vi "Main.vi"() -> ()   [LabVIEW 2025, in "Application.lvlib"]
uses:
  Application.lvlib
  Application Data--cluster.ctl
  State--enum.ctl
  <vilib>/Utility/error.llb/DialogType.ctl
  Logging - Text/Logging - Text.lvlib
  AI DAQ/AI DAQ.lvlib
panel:
  out "Waveform Graph":waveform(dbl)[](graph)
  in  "Start Acq and Log":bool
  in  "Logging File Path":path=path "C:/Users/David Corney/Documents/default log.txt"
  in  "AI DAQ Task Name":refnum<k21>="MyAnalogInTask_DiesEl"
  in  "About DQMH":bool
  out "Status":string
  out "version":string
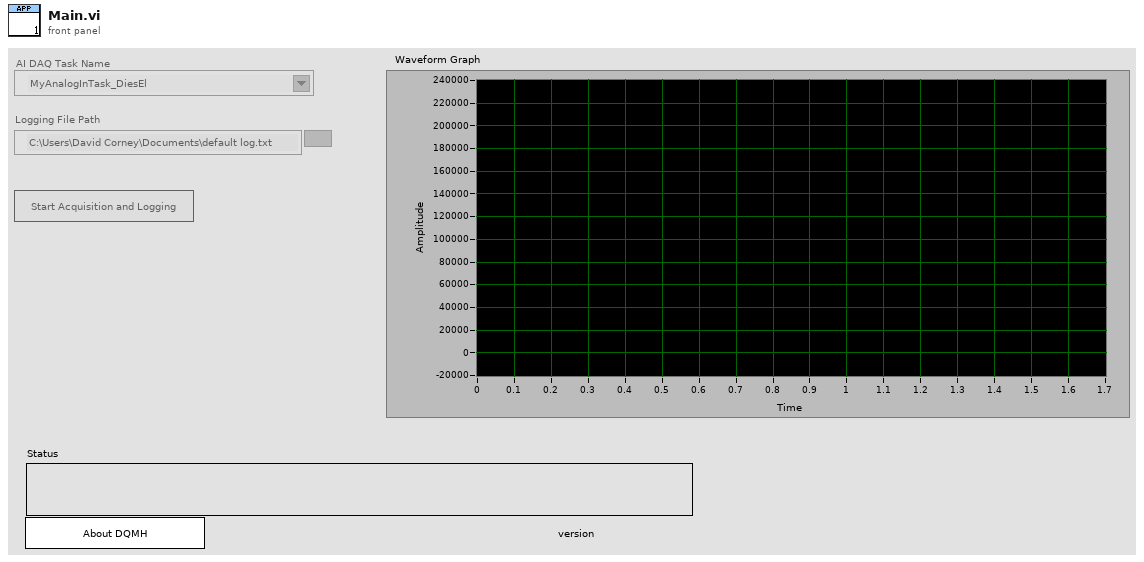
[diagram p1: front panel]
types:
  T1 = typedef "Application.lvlib/State--enum.ctl" = enum16{"Initialize", "Initialize Panel", "UI Interlocks", "Start Modules", "Update Status", "Wait for Event", "Exit"}
  T2 = typedef "Application.lvlib/Application Data--cluster.ctl" = cluster{"Status":string, "Singleton Controls":refnum<vi>[], "Cloneable Controls":refnum<vi>[], "App Controls":refnum<vi>[]}
  T3 = typedef "Logging - Text.lvlib/Broadcast Events--cluster.ctl" = cluster{"Module Did Init":refnum<user-event>, "Status Updated":refnum<user-event>, "Error Reported":refnum<user-event>, "Module Did Stop":refnum<user-event>, "Update Module Execution Status":refnum<user-event>}
  T4 = typedef "AI DAQ.lvlib/Broadcast Events--cluster.ctl" = cluster{"Module Did Init":refnum<user-event>, "Status Updated":refnum<user-event>, "Error Reported":refnum<user-event>, "Module Did Stop":refnum<user-event>, "Update Module Execution Status":refnum<user-event>, "AI DAQ WF Data":refnum<user-event>}
  T5 = enum8{"Enabled", "Disabled", "Disabled and Grayed Out"}
  T6 = typedef "DialogType.ctl" = u16
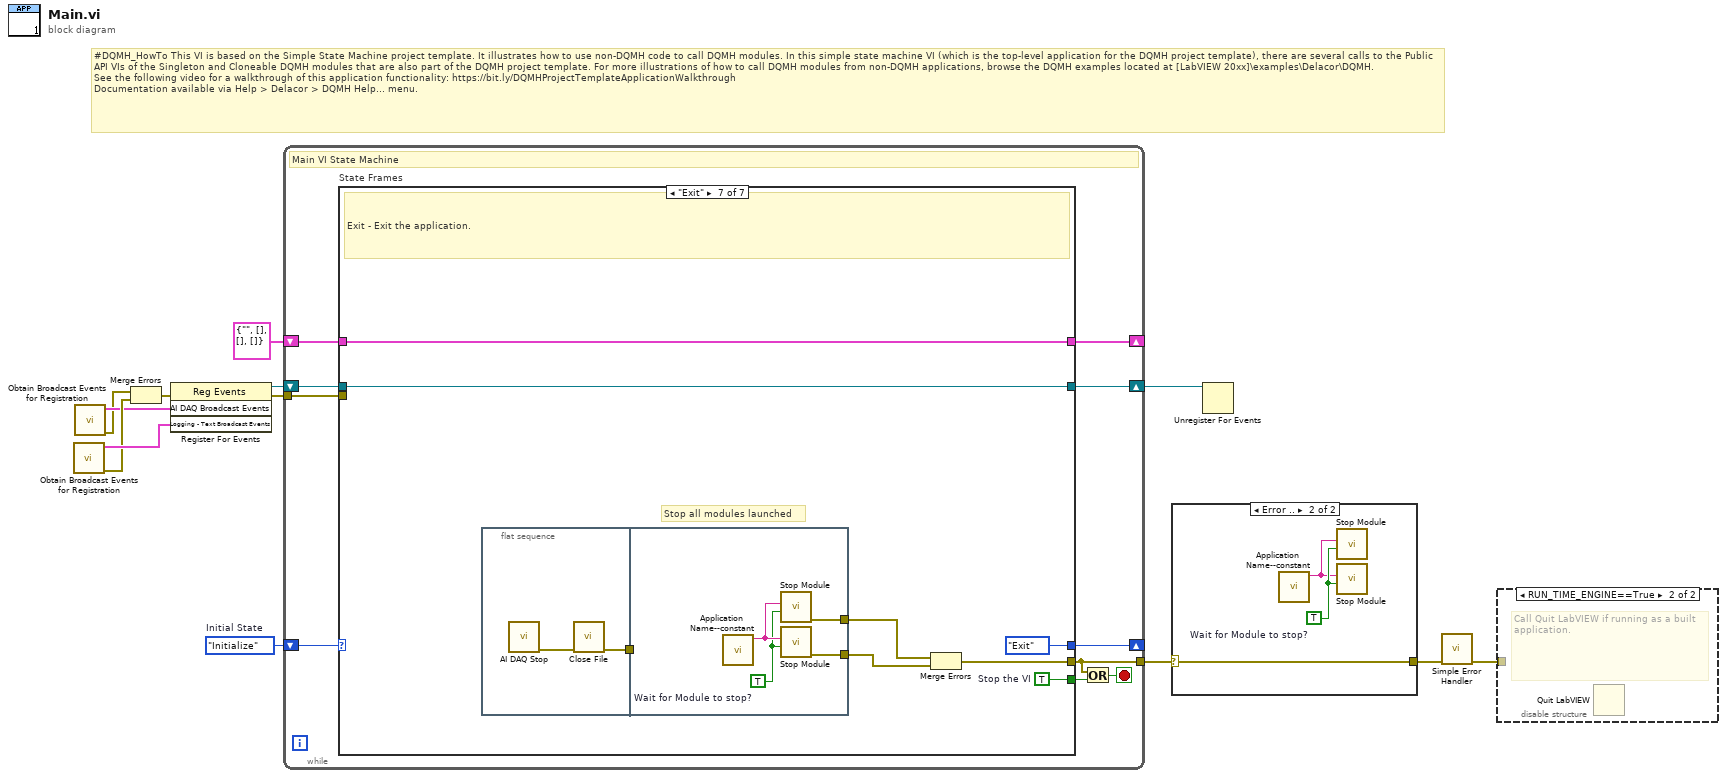
[diagram p0: block diagram]
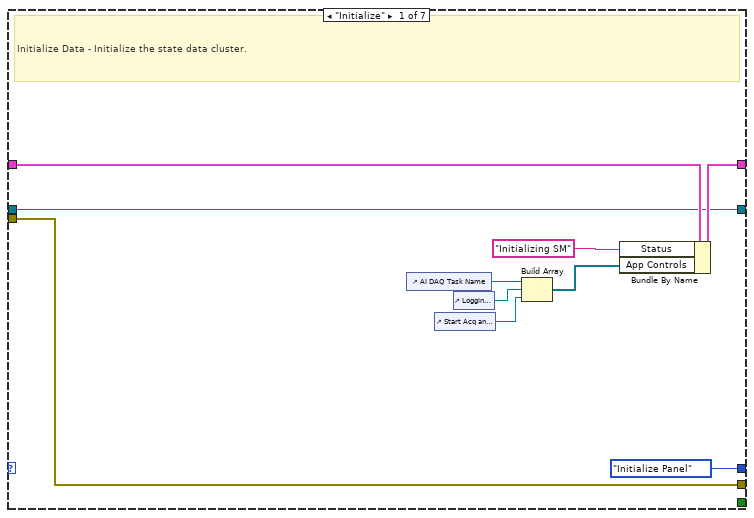
[diagram p3: hidden frame]
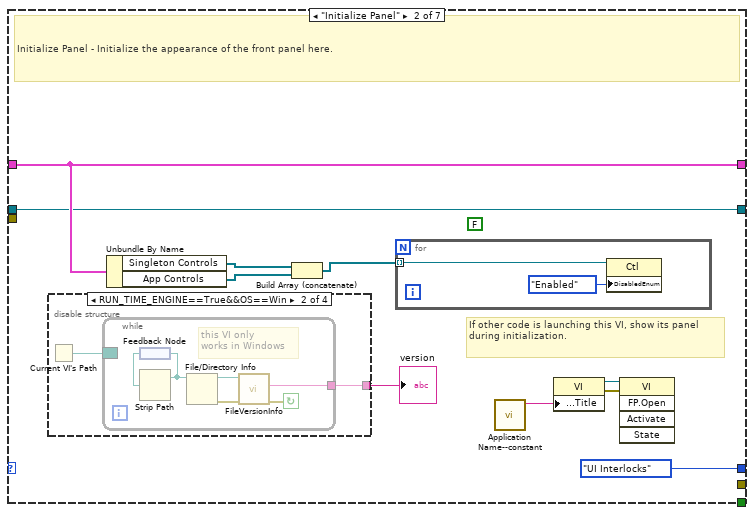
[diagram p4: hidden frame]
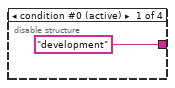
[diagram p5: hidden frame]
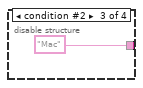
[diagram p6: hidden frame]
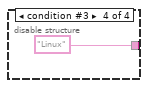
[diagram p7: hidden frame]
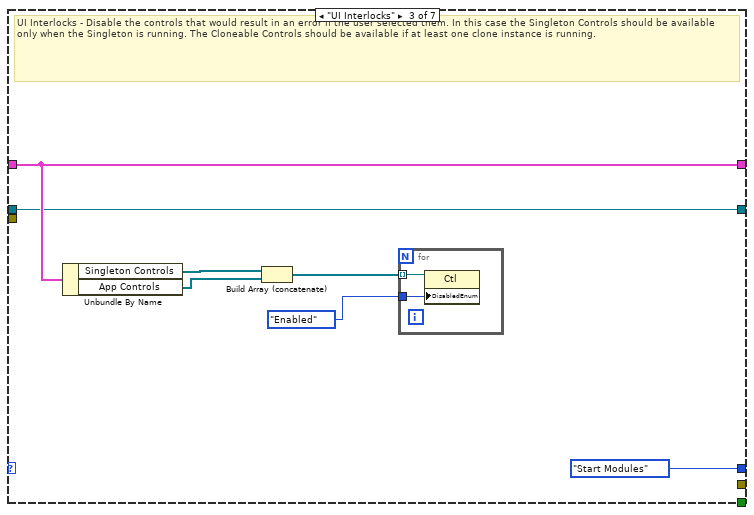
[diagram p8: hidden frame]
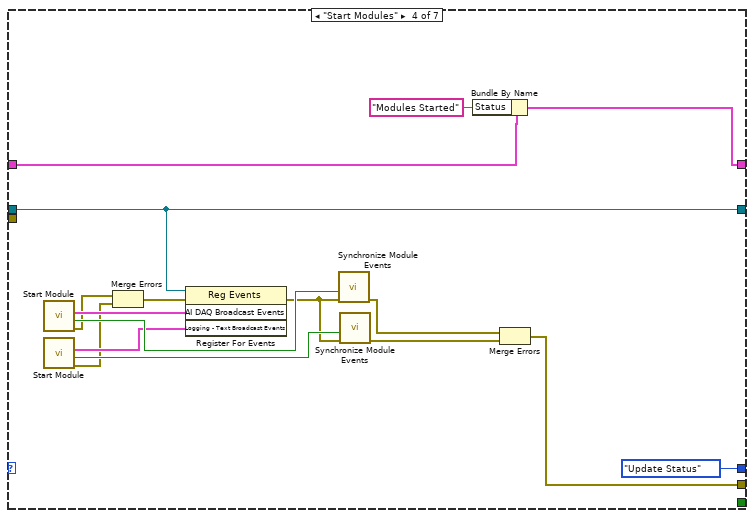
[diagram p9: hidden frame]
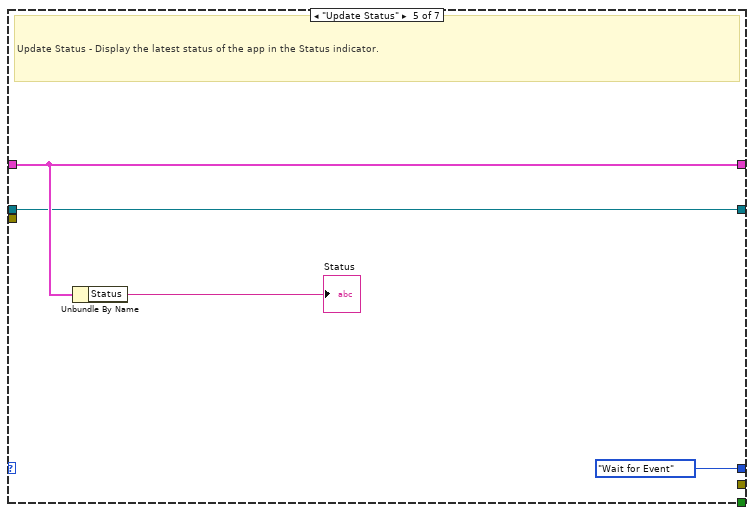
[diagram p10: hidden frame]
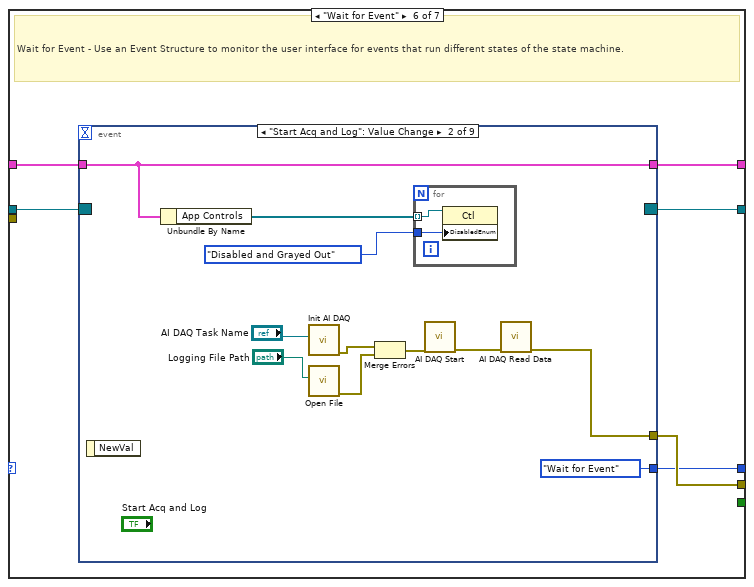
[diagram p11: hidden frame]
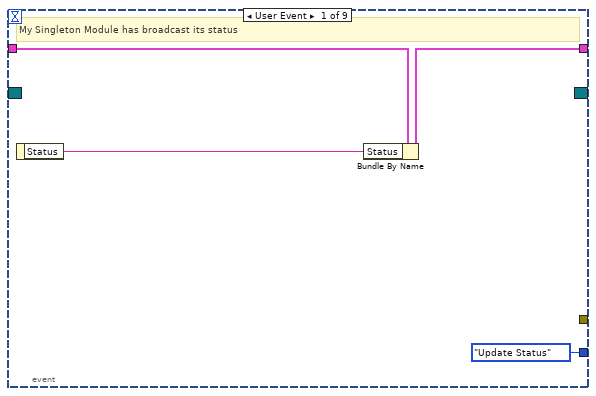
[diagram p12: hidden frame]
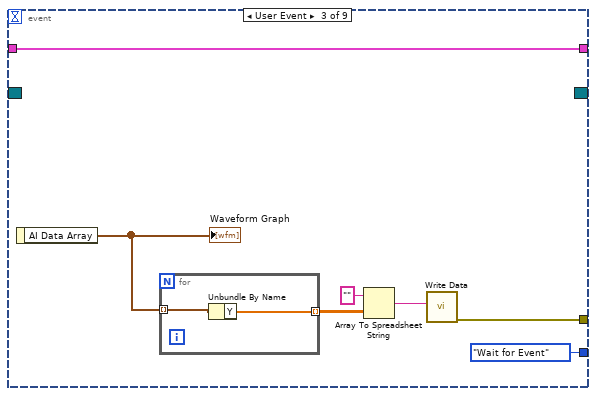
[diagram p13: hidden frame]
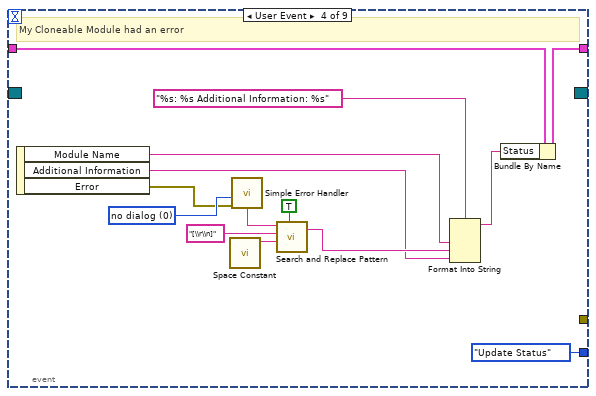
[diagram p14: hidden frame]
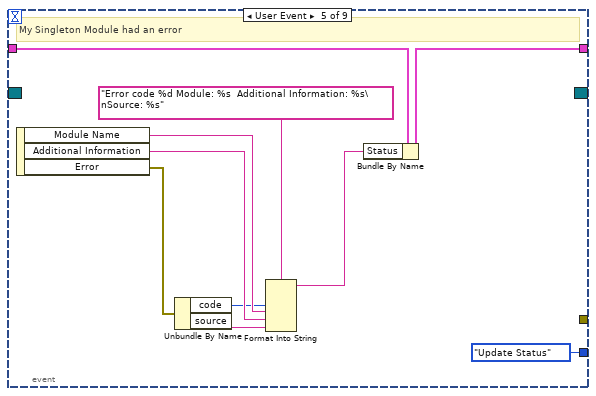
[diagram p15: hidden frame]
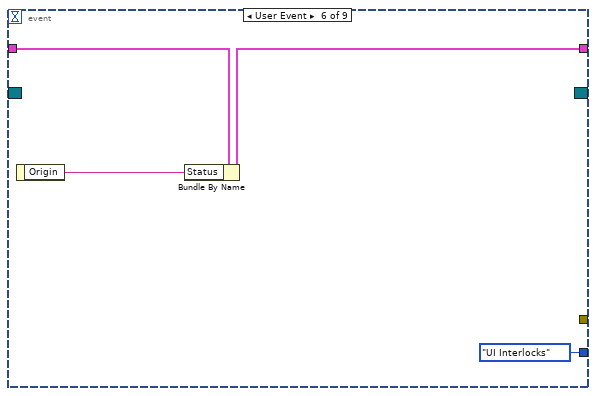
[diagram p16: hidden frame]
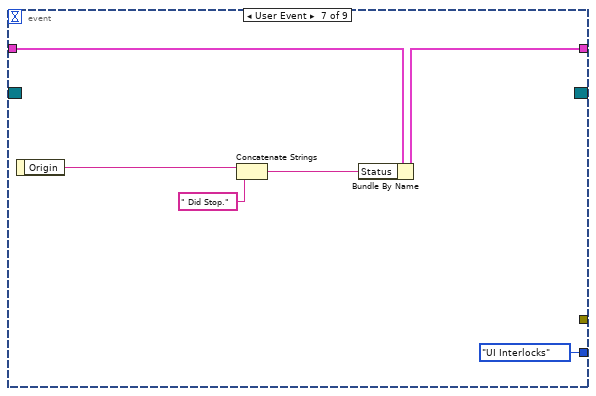
[diagram p17: hidden frame]
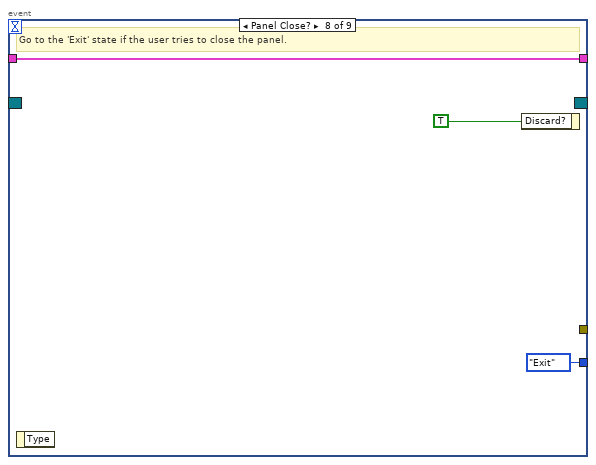
[diagram p18: hidden frame]
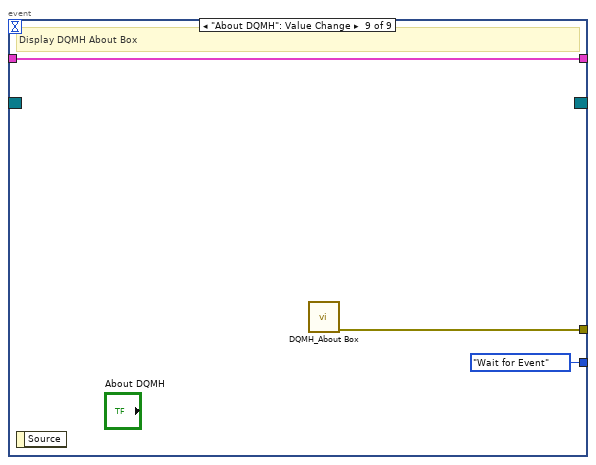
[diagram p19: hidden frame]
diagram:
  w9 = State--enum."Initialize"  # Initial State
  # "#DQMH_HowTo This VI is based on the Simple State Machine project template. It illustrates how to use non-DQMH code to call DQMH modules. In this simple state machine VI (which is the top-level application for the DQMH project template), there are several calls to the Public API VIs of the Singleton and Cloneable DQMH modules that are also part of the DQMH project template. For more illustrations of how to call DQMH modules from non-DQMH applications, browse the DQMH examples located at [LabVIEW 20xx]\\examples\\Delacor\\DQMH.\nSee the following video for a walkthrough of this application functionality: https://bit.ly/DQMHProjectTemplateApplicationWalkthrough\nDocumentation available via Help > Delacor > DQMH Help... menu."
  n1 = call "Obtain Broadcast Events for Registration.vi"() -> ("error out"=w5:errorcluster, "Logging - Text Broadcast Events"=w6:T3)  [unwired: 9 in, 1 out]
  n2 = call "Obtain Broadcast Events for Registration.vi"() -> ("error out"=w3:errorcluster, "AI DAQ Broadcast Events"=w4:T4)  [unwired: 9 in, 1 out]
  n3 = Merge Errors(w3, w5) -> (w11:errorcluster)
  n4 = register-events(error in=w11, w4, w6) -> (reference out=w8:refnum<event-registration>, error out=w12:errorcluster)  [unwired: 1 in]
  n5 = while {
    shift-right: [w20] -> _
    shift-left: T2 {"Status"="", "Singleton Controls"=[], "Cloneable Controls"=[], "App Controls"=[]} ("Data Cluster") -> [w21]
    tunnel: [w23] -> w2
    shift-right: [w16] -> _
    shift-left: w9 -> [w18]
    shift-right: [w14] -> w7
    shift-left: w8 -> [w15]
    tunnel: w12 -> [w22]
    stop <- w17 stop-if-true
    # "Main VI State Machine"
    n6 = case "State Frames" shown="\"Exit\"" w18 {
      tunnel: [w33 _ _ w71 _ w91 w165] -> w23
      tunnel: w21 -> [w32 w42 w63 w68 w85 w88 w164]
      tunnel: [w31 w42 w63 w66 w85 w87 w164] -> w20
      tunnel: [_ _ _ _ _ _ w163] -> w19
      tunnel: [State--enum."Initialize Panel" ("State") State--enum."UI Interlocks" ("State") State--enum."Start Modules" ("State") State--enum."Update Status" ("State") State--enum."Wait for Event" ("State") w86 State--enum."Exit" ("State")] -> w16
      tunnel: w15 -> [w28 w40 w61 w80 w82 w90 w161]
      tunnel: [w28 w40 w61 w80 w82 w89 w161] -> w14
      tunnel: w22 -> [w33 _ _ _ _ _ _]
      frame "Initialize" {
        # "Initialize Data - Initialize the state data cluster."
        n7 = control-ref of="AI DAQ Task Name"() -> (w26:refnum<vi>)
        n8 = control-ref of="Start Acq and Log"() -> (w24:refnum<vi>)
        n9 = control-ref of="Logging File Path"() -> (w25:refnum<vi>)
        n10 = Build Array(w26, w25, w24) -> (w27:refnum<vi>[])
        n11 = Bundle By Name(cluster=w32, "Status"="Initializing SM" ("Initial Message"), "App Controls"=w27) -> (w31:T2)
      }
      frame "Initialize Panel" {
        (unwired) FALSE ("My Singleton Module Init?")
        # "If other code is launching this VI, show its panel during initialization."
        # "Initialize Panel - Initialize the appearance of the front panel here."
        n12 = disable-structure "Conditional Disable Structure" shown="RUN_TIME_ENGINE==True&&OS==Win" {
          disable-tunnel: ["development" w45 "Mac" "Linux"] -> w39
          frame condition #0 (active) {
          }
          frame condition #1 {
            n13 = Current VI's Path() -> (path=w46:path)
            n14 = while {
              border: w46 -> [_]
              tunnel: [w47] -> w45
              stop <- w51 continue-if-true
              # "this VI only \nworks in Windows"
              n15 = feedback #1() -> (w50:path)
              n16 = Strip Path(path=w50) -> (stripped path=w49:path)  [unwired: 1 out]
              n17 = feedback-in #1(w49) -> ()
              n18 = File/Directory Info(path=w49) -> (path out=w48:path, error out=w52:errorcluster)  [unwired: 1 in, 5 out]
              n19 = call <vilib>:"FileVersionInfo.vi"("error in (no error)"=w52, "Application Path in"=w48) -> ("error out"=w51:errorcluster, "File Version Info"=w47:string)  [unwired: 6 in, 2 out]
            }
          }
          frame condition #2 {
          }
          frame condition #3 {
          }
        }
        "version" <- w39
        n20 = Unbundle By Name(w42) -> ("Singleton Controls"=w36:refnum<vi>[], "App Controls"=w35:refnum<vi>[])
        n21 = Build Array (concatenate)(w36, w35) -> (w34:refnum<vi>[])
        n22 = for {
          tunnel: w34 -> [w56] mode=indexing
          n23 = property on="Property Node" class="Ctl"(reference=w56, "DisabledEnum"=T5."Enabled" ("Disabled")) -> ()  [unwired: 1 in, 2 out]
        }
        n24 = call "Application Name--constant.vi"() -> ("Application Name"=w38:string)  [unwired: 11 in]
        n25 = property on="Property Node" class="VI"("Front Panel.Title"=w38) -> (reference out=w37:refnum<vi>, error out=w43:errorcluster)  [unwired: 2 in]
        n26 = invoke class="VI" method="FP.Open"(reference=w37, error in=w43) -> ()  [unwired: 3 in, 5 out]
      }
      frame "UI Interlocks" {
        # "UI Interlocks - Disable the controls that would result in an error if the user selected them. In this case the Singleton Controls should be available only when the Singleton is running. The Cloneable Controls should be available if at least one clone instance is running."
        n27 = Unbundle By Name(w63) -> ("Singleton Controls"=w60:refnum<vi>[], "App Controls"=w57:refnum<vi>[])
        n28 = Build Array (concatenate)(w60, w57) -> (w59:refnum<vi>[])
        n29 = for {
          tunnel: w59 -> [w65] mode=indexing
          tunnel: T5."Enabled" ("Disabled") -> [w64]
          n30 = property on="Property Node" class="Ctl"(reference=w65, "DisabledEnum"=w64) -> ()  [unwired: 1 in, 2 out]
        }
      }
      frame "Start Modules" {
        n31 = call "Start Module.vi"() -> ("error out"=w75:errorcluster, "Wait for Event Sync?"=w78:bool, "AI DAQ Broadcast Events"=w79:T4)  [unwired: 8 in, 1 out]
        n32 = call "Start Module.vi"() -> ("error out"=w74:errorcluster, "Wait for Event Sync?"=w76:bool, "Logging - Text Broadcast Events"=w77:T3)  [unwired: 8 in, 1 out]
        n33 = Merge Errors(w75, w74) -> (w73:errorcluster)
        n34 = register-events(reference=w80, error in=w73, w79, w77) -> (error out=w72:errorcluster)  [unwired: 1 out]
        n35 = call "Synchronize Module Events.vi"("error in"=w72, "Wait for Event Sync?"=w78) -> ("error out"=w70:errorcluster)  [unwired: 9 in]
        n36 = call "Synchronize Module Events.vi"("error in"=w72, "Wait for Event Sync?"=w76) -> ("error out"=w69:errorcluster)  [unwired: 9 in]
        n37 = Bundle By Name(cluster=w68, "Status"="Modules Started") -> (w66:T2)
        n38 = Merge Errors(w70, w69) -> (w71:errorcluster)
      }
      frame "Update Status" {
        # "Update Status - Display the latest status of the app in the Status indicator."
        n39 = Unbundle By Name(w85) -> ("Status"=→"Status":string)
      }
      frame "Wait for Event" {
        # "Wait for Event - Use an Event Structure to monitor the user interface for events that run different states of the state machine."
        n40 = event shown="[1] \"Start Acq and Log\": Value Change" {
          selector: w90 -> [_ _ _ _ _ _ _ _ _]
          dyn-events: [_ _ _ _ _ _ _ _ _] -> w89
          timeout: _ -> [_ _ _ _ _ _ _ _ _]
          tunnel: [_ w104 w110 _ _ _ _ _ w155] -> w91
          tunnel: [w93 w103 w115 w130 w139 w142 w149 w153 w157] -> w87
          tunnel: w88 -> [w94 w103 w115 w131 w140 w144 w150 w153 w157]
          tunnel: [State--enum."Update Status" ("State") State--enum."Wait for Event" ("State") State--enum."Wait for Event" ("State") State--enum."Update Status" ("State") State--enum."Update Status" ("State") State--enum."UI Interlocks" ("State") State--enum."UI Interlocks" ("State") State--enum."Exit" ("State") State--enum."Wait for Event" ("State")] -> w86
          event User Event {
            # "My Singleton Module has broadcast its status"
            n41 = event-data() -> ("Status"=w95:string)  [unwired: 1 in]
            n42 = Bundle By Name(cluster=w94, "Status"=w95) -> (w93:T2)
          }
          event "Start Acq and Log": Value Change {
            n43 = event-data() -> ()  [unwired: 1 in, 1 out]
            n44 = Unbundle By Name(w103) -> ("App Controls"=w96:refnum<vi>[])
            n45 = call "Init AI DAQ.vi"("AI DAQ Task Name"="AI DAQ Task Name") -> ("error out"=w98:errorcluster)  [unwired: 10 in]
            n46 = call "Open File.vi"("Path"="Logging File Path") -> ("error out"=w97:errorcluster)  [unwired: 10 in]
            n47 = Merge Errors(w98, w97) -> (w99:errorcluster)
            n48 = for {
              tunnel: T5."Disabled and Grayed Out" ("Disabled") -> [w108]
              tunnel: w96 -> [w107] mode=indexing
              n49 = property class="Ctl"(reference=w107, "DisabledEnum"=w108) -> ()  [unwired: 1 in, 2 out]
            }
            n50 = call "AI DAQ Start.vi"("error in"=w99) -> ("error out"=w105:errorcluster)  [unwired: 10 in]
            n51 = call "AI DAQ Read Data.vi"("error in"=w105) -> ("error out"=w104:errorcluster)  [unwired: 9 in, 1 out]
          }
          event User Event {
            n52 = event-data() -> ("AI Data Array"=w113:waveform(dbl)[])  [unwired: 1 in]
            "Waveform Graph" <- w113
            n53 = for {
              tunnel: w113 -> [w117] mode=indexing
              tunnel: [w116] -> w112 mode=indexing
              n54 = Unbundle By Name(w117) -> ("Y"=w116:dbl[])
            }
            n55 = Array To Spreadsheet String(array=w112, 3:"" ("format string")) -> (spreadsheet string=w111:string)  [unwired: 1 in]
            n56 = call "Write Data.vi"("Text Data"=w111) -> ("error out"=w110:errorcluster)  [unwired: 10 in]
          }
          event User Event {
            w122 = T6 0 items=["no dialog", "OK message", "continue or stop message", "OK message + warnings", "continue/stop + warnings"] ("type of dialog (OK msg:1)")
            # "My Cloneable Module had an error"
            n57 = event-data() -> ("Module Name"=w119:string, "Additional Information"=w120:string, "Error"=w121:errorcluster)  [unwired: 1 in]
            n58 = call <vilib>:"Space Constant.vi"() -> ("String"=w126:string)
            n59 = call <vilib>:"Simple Error Handler.vi"("type of dialog (OK msg:1)"=w122, "error in (no error)"=w121) -> ("message"=w123:string)  [unwired: 3 in, 4 out]
            n60 = call <vilib>:"Search and Replace Pattern.vi"("string"=w123, "regular expression (\"\")"="[\\r\\n]" ("regular expression (\"\")"), "replace string (\"\")"=w126, "replace all? (F)"=TRUE ("replace all CR/LF with spaces")) -> ("result string"=w124:string)  [unwired: 1 in, 1 out]
            n61 = Format Into String(format string="%s: %s Additional Information: %s", w119, w124, w120) -> (resulting string=w118:string)  [unwired: 2 in, 1 out]
            n62 = Bundle By Name(cluster=w131, "Status"=w118) -> (w130:T2)
          }
          event User Event {
            # "My Singleton Module had an error"
            n63 = event-data() -> ("Module Name"=w133:string, "Additional Information"=w137:string, "Error"=w141:errorcluster)  [unwired: 1 in]
            n64 = Unbundle By Name(w141) -> ("code"=w132:i32, "source"=w136:string)
            n65 = Format Into String(format string="Error code %d Module: %s  Additional Information: %s\nSource: %s", w132, w133, w137, w136) -> (resulting string=w134:string)  [unwired: 2 in, 1 out]
            n66 = Bundle By Name(cluster=w140, "Status"=w134) -> (w139:T2)
          }
          event User Event {
            n67 = event-data() -> ("Origin"=w143:string)  [unwired: 1 in]
            n68 = Bundle By Name(cluster=w144, "Status"=w143) -> (w142:T2)
          }
          event User Event {
            n69 = event-data() -> ("Origin"=w147:string)  [unwired: 1 in]
            n70 = Concatenate Strings(w147, " Did Stop.") -> (w146:string)
            n71 = Bundle By Name(cluster=w150, "Status"=w146) -> (w149:T2)
          }
          event Panel Close? {
            # "Go to the 'Exit' state if the user tries to close the panel."
            n72 = event-data() -> ()  [unwired: 1 in, 1 out]
            n73 = event-data ("Event Filter Node")("Discard?"=TRUE) -> ()  [unwired: 1 in, 1 out]
          }
          event "About DQMH": Value Change {
            # "Display DQMH About Box"
            n74 = event-data() -> ()  [unwired: 1 in, 1 out]
            n75 = call <vilib>:"DQMH_About Box.vi"() -> ("error out"=w155:errorcluster)  [unwired: 11 in]
          }
        }
      }
      frame "Exit" {
        w163 = TRUE  # Stop the VI
        # "Stop all modules launched"
        # "Exit - Exit the application."
        n76 = flat-sequence {
          tunnel: [w166] -> w158
          tunnel: [w169] -> w159
          tunnel: [w168] -> w160
          tunnel: w158 -> [_]
          frame #0 {
            n77 = call "AI DAQ Stop.vi"() -> ("error out"=w167:errorcluster)  [unwired: 11 in]
            n78 = call "Close File.vi"("error in"=w167) -> ("error out"=w166:errorcluster)  [unwired: 10 in]
          }
          frame #1 {
            w170 = TRUE  # Wait for Module to stop?
            n79 = call "Application Name--constant.vi"() -> ("Application Name"=w171:string)  [unwired: 11 in]
            n80 = call "Stop Module.vi"("Wait for Module to Stop? (F)"=w170, "Origin"=w171) -> ("error out"=w169:errorcluster)  [unwired: 9 in]
            n81 = call "Stop Module.vi"("Wait for Module to Stop? (F)"=w170, "Origin"=w171) -> ("error out"=w168:errorcluster)  [unwired: 9 in]
          }
        }
        n82 = Merge Errors(w159, w160) -> (w165:errorcluster)
      }
    }
    n83 = Or(x=w23, y=w19) -> (x .or. y?=w17:bool)
  }
  n84 = case shown="Error .." w2 {
    selector: w2 -> [w172 w173]
    tunnel: [w172 w173] -> w1
    frame No Error {
    }
    frame Error {
      w175 = TRUE  # Wait for Module to stop?
      n85 = call "Application Name--constant.vi"() -> ("Application Name"=w174:string)  [unwired: 11 in]
      n86 = call "Stop Module.vi"("Wait for Module to Stop? (F)"=w175, "Origin"=w174) -> ()  [unwired: 9 in, 1 out]
      n87 = call "Stop Module.vi"("Wait for Module to Stop? (F)"=w175, "Origin"=w174) -> ()  [unwired: 9 in, 1 out]
    }
  }
  n88 = Unregister For Events(event registration refnum=w7) -> ()  [unwired: 1 in, 1 out]
  n89 = call <vilib>:"Simple Error Handler.vi"("error in (no error)"=w1) -> ("error out"=w13:errorcluster)  [unwired: 4 in, 4 out]
  n90 = disable-structure "Conditional Disable Structure" shown="RUN_TIME_ENGINE==True" {
    disable-tunnel: w13 -> [_ _]
    frame condition #0 (active) {
    }
    frame condition #1 {
      # "Call Quit LabVIEW if running as a built application."
      n91 = Quit LabVIEW() -> ()  [unwired: 1 in]
    }
  }
